vi "Read Adjacency List.vi"(8 "error in (no error)":errorcluster, 11 "Graph in":refnum<class "Graph.lvclass">) -> (0 "error out":errorcluster, 2 "Adjacency List":map{string, string[]}(c390), 3 "Graph out":refnum<class "Graph.lvclass">)   [LabVIEW 2025, in "AOC.lvlib" / "Graph.lvlib" / "Graph.lvclass"]
uses:
  Graph.lvclass
  Graph.lvclass/Graph.ctl
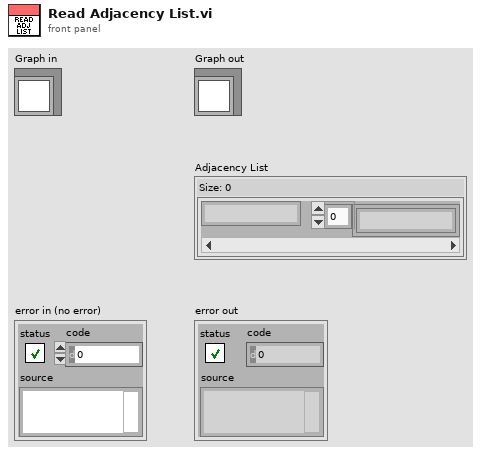
[diagram p1: front panel]
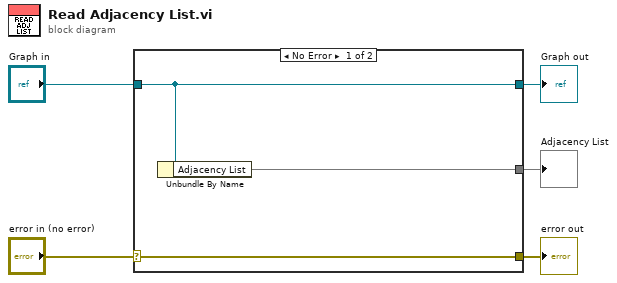
[diagram p0: block diagram]
diagram:
  n1 = case shown="No Error" "error in (no error)" {
    selector: "error in (no error)" -> [w8 w9]
    tunnel: [w8 w9] -> w4
    tunnel: [w7 w10] -> w2
    tunnel: "Graph in" -> [w7 w10]
    tunnel: [w6 _] -> w1
    frame No Error {
      n2 = Unbundle By Name(w7) -> ("Adjacency List"=w6:map{string, string[]})
    }
    frame Error {
    }
  }
  "error out" <- w4
  "Graph out" <- w2
  "Adjacency List" <- w1
